vi "Remove Duplicates from 1D Array (I8)__ogtk.vi"(0 "Input Array":i8[](array[numeric])) -> (1 "Output Array":i8[](array[numeric]), 2 "indices of removed elements":i32[](array[numeric]))   [LabVIEW 2011]
doc: "This polymorphic VI removes all duplicate elements in <B>Input Array</B> and outputs the result as <B>Output Array</B>. It also outputs the <B>indices of removed elements<B>."
panel:
  # "Remove Duplicates from 1D Array.vi\n\nRemoves duplicate array elements and returns the indices of the removed elements\n\nPlease visit http://www.OpenG.org to learn about the\nOpen Source LabVIEW software movement.\n\nNOTICE -- YOU MUST LEAVE THIS NOTICE IN PLACE.  PER THE TERMS OF THE LICENSE BELOW, YOU MAY SUBLICENSE THIS SOFTWARE \nIN ANY WAY THAT DOES NOT CONFLICT WITH THIS LICENSE.\n\n### BSD License (http://www.opensource.org/licenses/bsd-license.php) Begin ###\n \nCopyright (c) 2002, Jim Kring <jim@jimkring.com>\n\nAll rights reserved.\n\nRedistribution and use in source and binary forms, with or without modification, are permitted provided that the following conditions are met:\n\n    * Redistributions of source code must retain the above copyright notice, this list of conditions and the following disclaimer.\n    * Redistributions in binary form must reproduce the above copyright notice, this list of conditions and the following disclaimer in the \n       documentation and/or other materials provided with the distribution.\n    * Neither the name of SciWare, James Kring, Inc., nor the names of its contributors may be used to endorse or promote products derived \n       from this software without specific prior written permission.\n\nTHIS SOFTWARE IS PROVIDED BY THE COPYRIGHT HOLDERS AND CONTRIBUTORS \"AS IS\" AND ANY EXPRESS OR IMPLIED WARRANTIES, \nINCLUDING, BUT NOT LIMITED TO, THE IMPLIED WARRANTIES OF MERCHANTABILITY AND FITNESS FOR A PARTICULAR PURPOSE ARE \nDISCLAIMED. IN NO EVENT SHALL THE COPYRIGHT OWNER OR CONTRIBUTORS BE LIABLE FOR ANY DIRECT, INDIRECT, INCIDENTAL,\n SPECIAL, EXEMPLARY, OR CONSEQUENTIAL DAMAGES (INCLUDING, BUT NOT LIMITED TO, PROCUREMENT OF SUBSTITUTE GOODS OR \nSERVICES; LOSS OF USE, DATA, OR PROFITS; OR BUSINESS INTERRUPTION) HOWEVER CAUSED AND ON ANY THEORY OF LIABILITY, \nWHETHER IN CONTRACT, STRICT LIABILITY, OR TORT (INCLUDING NEGLIGENCE OR OTHERWISE) ARISING IN ANY WAY OUT OF THE USE \nOF THIS SOFTWARE, EVEN IF ADVISED OF THE POSSIBILITY OF SUCH DAMAGE.\n\n### BSD License End ###"
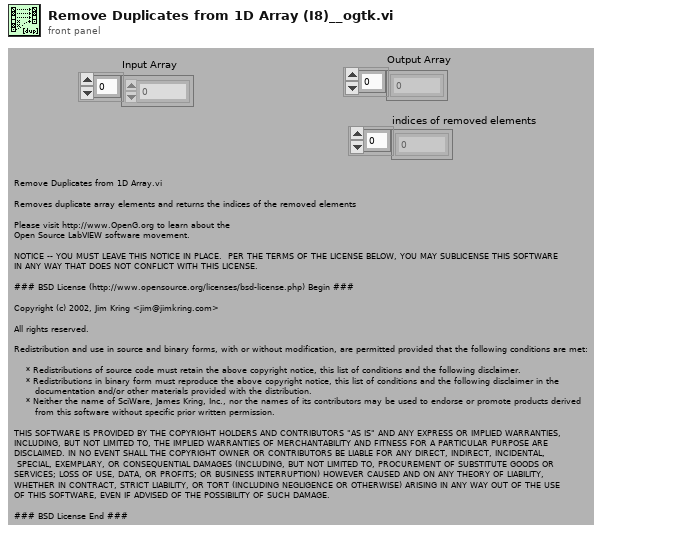
[diagram p1: front panel]
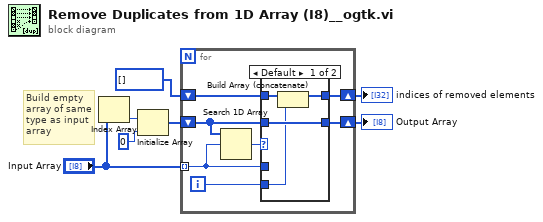
[diagram p0: block diagram]
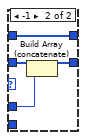
[diagram p2: hidden frame]
diagram:
  # "Build empty array of same type as input array"
  n1 = Index Array(array="Input Array") -> (element=w3:i8)  [unwired: 1 in]
  n2 = Initialize Array(w3, 0 ("Dimension Size")) -> (w2:i8[])
  n3 = for {
    tunnel: "Input Array" -> [w13] mode=indexing
    shift-right: [w12] -> w6
    shift-left: w2 -> [w11]
    shift-right: [w9] -> w4
    shift-left: i32[] [] -> [w8]
    i -> [w10]
    n4 = Search 1D Array(1D array=w11, element=w13) -> (index of element=w14:i32)  [unwired: 1 in]
    n5 = case shown="Default" w14 {
      tunnel: w13 -> [_ w22]
      tunnel: [w18 w20] -> w12
      tunnel: w11 -> [w18 w21]
      tunnel: w10 -> [w15 _]
      tunnel: [w16 w19] -> w9
      tunnel: w8 -> [w17 w19]
      frame Default {
        n6 = Build Array (concatenate)(w17, w15) -> (w16:i32[])
      }
      frame -1 {
        n7 = Build Array (concatenate)(w21, w22) -> (w20:i8[])
      }
    }
  }
  "Output Array" <- w6
  "indices of removed elements" <- w4
